vi "Test Actor.vi"() -> ()   [LabVIEW 2018]
uses:
  Scripting/Actor/State.ctl
  Scripting/Actor.lvclass
  Scripting/Interface.lvclass/Interface.ctl
  <vilib>/Utility/error.llb/Clear Errors.vi
  Scripting/Interface.lvclass
panel:
  in  "Stop":bool
  in  "Get State":bool
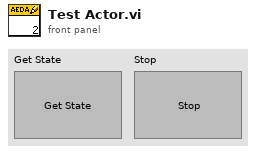
[diagram p1: front panel]
types:
  T1 = cluster{"Current State":refnum<event-registration>, "Actor Stopped":refnum<event-registration>, "Current State":refnum<event-registration>}
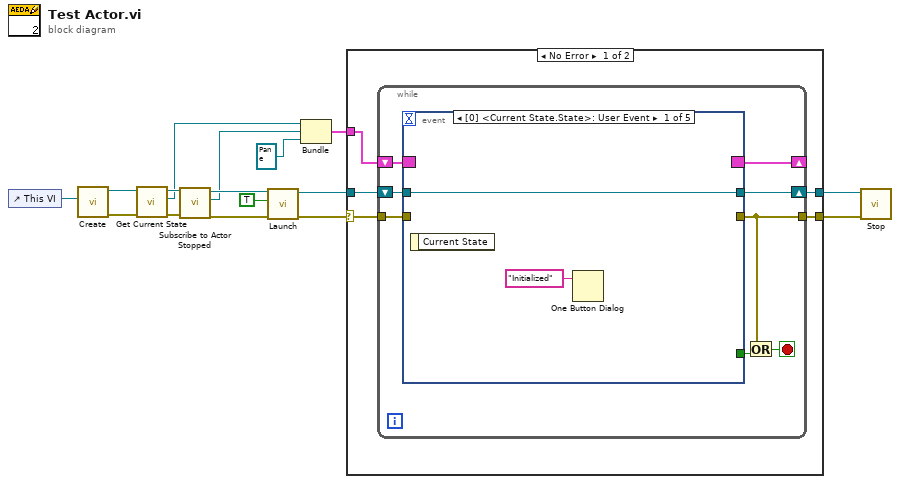
[diagram p0: block diagram]
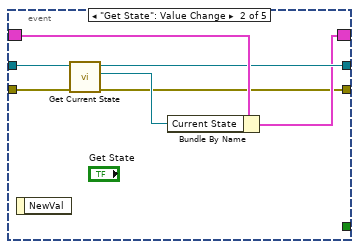
[diagram p2: hidden frame]
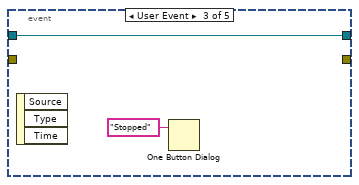
[diagram p3: hidden frame]
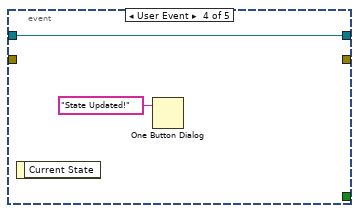
[diagram p4: hidden frame]
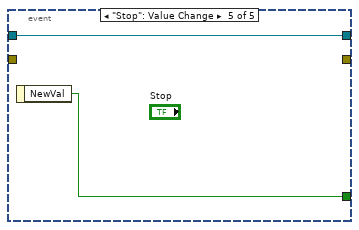
[diagram p5: hidden frame]
diagram:
  n1 = control-ref of="This VI"() -> (w12:refnum<vi>)
  n2 = call "Create.vi"("Owner"=w12) -> ("error out"=w4:errorcluster, "API out"=w5:refnum<class "Interface.lvclass">)  [unwired: 9 in]
  n3 = call "Get Current State.vi"("error in (no error)"=w4, "API In"=w5) -> ("error out"=w3:errorcluster, "Current State"=w1:refnum<event-registration>, "API out"=w2:refnum<class "Interface.lvclass">)  [unwired: 6 in, 1 out]
  n4 = call "Subscribe to Actor Stopped.vi"("error in (no error)"=w3, "API in"=w2) -> ("error out"=w15:errorcluster, "Actor Stopped"=w14:refnum<event-registration>, "API out"=w16:refnum<class "Interface.lvclass">)  [unwired: 7 in]
  n5 = call "Launch.vi"("error in (no error)"=w15, "Show Front Panel? (F)"=TRUE, "API in"=w16) -> ("error out"=w8:errorcluster, "API out"=w11:refnum<class "Interface.lvclass">)  [unwired: 6 in, 1 out]
  n6 = Bundle("Current State"=w1, "Actor Stopped"=w14, "Current State"=refnum<event-registration> refnum) -> (w13:T1)  [unwired: 1 in]
  n7 = case shown="No Error" w8 {
    selector: w8 -> [w18 w45]
    tunnel: w13 -> [w17 _]
    tunnel: w11 -> [w21 w46]
    tunnel: [w20 w46] -> w6
    tunnel: [w19 w45] -> w7
    frame No Error {
      n8 = while {
        shift-right: [w28] -> _
        shift-left: w17 -> [w29]
        shift-right: [w26] -> w20
        shift-left: w21 -> [w27]
        tunnel: [w23] -> w19
        tunnel: w18 -> [w22]
        stop <- w24 stop-if-true
        n9 = event shown="[0] <Current State.State>: User Event" {
          selector: w29 -> [_ w36 _ _ _]
          dyn-events: [_ w34 _ _ _] -> w28
          timeout: _ -> [_ _ _ _ _]
          tunnel: w27 -> [w30 w38 w40 w41 w43]
          tunnel: [w30 w35 w40 w41 w43] -> w26
          tunnel: [_ _ _ _ w44] -> w25
          tunnel: [_ w33 _ _ _] -> w23
          tunnel: w22 -> [_ w32 _ _ _]
          event User Event {
            n10 = event-data() -> ()  [unwired: 1 in, 1 out]
            n11 = One Button Dialog(message="Initialized") -> ()  [unwired: 1 in, 1 out]
          }
          event "Get State": Value Change {
            n12 = event-data() -> ()  [unwired: 1 in, 1 out]
            n13 = call "Get Current State.vi"("error in (no error)"=w32, "API In"=w38) -> ("error out"=w33:errorcluster, "Current State"=w37:refnum<event-registration>, "API out"=w35:refnum<class "Interface.lvclass">)  [unwired: 6 in, 1 out]
            n14 = Bundle By Name(cluster=w36, "Current State"=w37) -> (w34:T1)
          }
          event User Event {
            n15 = event-data() -> ()  [unwired: 1 in, 3 out]
            n16 = One Button Dialog(message="Stopped") -> ()  [unwired: 1 in, 1 out]
          }
          event User Event {
            n17 = event-data() -> ()  [unwired: 1 in, 1 out]
            n18 = One Button Dialog(message="State Updated!") -> ()  [unwired: 1 in, 1 out]
          }
          event "Stop": Value Change {
            n19 = event-data() -> ("NewVal"=w44:bool)  [unwired: 1 in]
          }
        }
        n20 = Or(x=w23, y=w25) -> (x .or. y?=w24:bool)
      }
    }
    frame Error {
    }
  }
  n21 = call "Stop.vi"("error in (no error)"=w7, "API out"=w6) -> ()  [unwired: 7 in, 3 out]
